vi "Send Inline Buffer.vi"(8 "error in (no error)":errorcluster, 10 "Inline Buffer Parameters":T1, 11 "Dispatcher Interface in":refnum<class "Dispatcher Interface.lvclass">) -> (0 "error out":errorcluster, 3 "Dispatcher Interface out":refnum<class "Dispatcher Interface.lvclass">)   [LabVIEW 2017, in "DSF Core.lvlib" / "Dispatcher Interface.lvclass"]
uses:
  Dispatcher Interface.lvclass
  C:/Git/DSF/Data Sharing Framework/Source/Core/Classes/Interfaces/Interface/Interface.lvclass
  Inline Buffer Parameters.ctl
  Command Data.ctl
  Command.ctl
  Parameters.ctl
  Interface/Interface.lvclass/Interface.ctl
  Response.ctl
  Write Dispatcher Command.vi
  Interface/Send Command.vi
  Interface/Write RT FIFO.vi
  Class Name.vi
  VIs/VI Name.vi
  Command Timeout.vi
  Read Dispatcher Response.vi
  Invalid Response Parameters.vi
  Invalid Response.vi
  Interface/Interface.lvclass
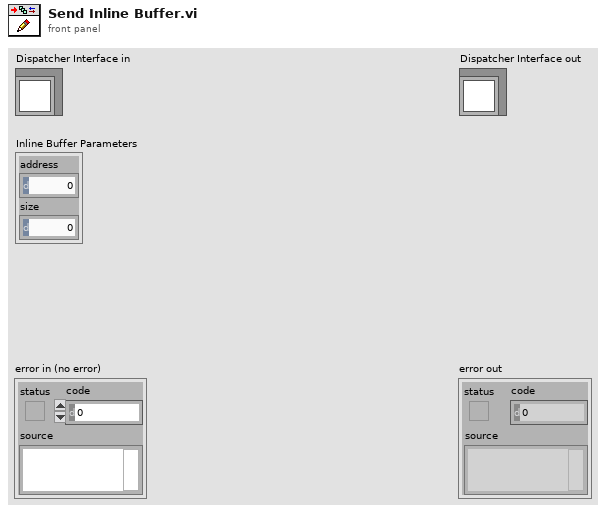
[diagram p1: front panel]
types:
  T1 = typedef "DSF Core.lvlib/Dispatcher Interface.lvclass/Inline Buffer Parameters.ctl" = cluster{"address":u64, "size":u64}
  T2 = typedef "DSF Core.lvlib/Dispatcher Interface.lvclass/Command.ctl" = enum8{"Rx", "Tx", "Set Inline Buffer", "Shutdown"}
  T3 = typedef "DSF Core.lvlib/Dispatcher Interface.lvclass/Parameters.ctl" = cluster{"arg1":u64, "arg2":u64}
  T4 = typedef "DSF Core.lvlib/Dispatcher Interface.lvclass/Command Data.ctl" = cluster{"Command":T2, "Parameters":T3}
  T5 = typedef "DSF Core.lvlib/Dispatcher Interface.lvclass/Response Data.ctl" = cluster{"Response":T6, "Parameters":T3}
  T6 = typedef "DSF Core.lvlib/Dispatcher Interface.lvclass/Response.ctl" = enum8{"General Ack", "Error", "Shutting Down"}
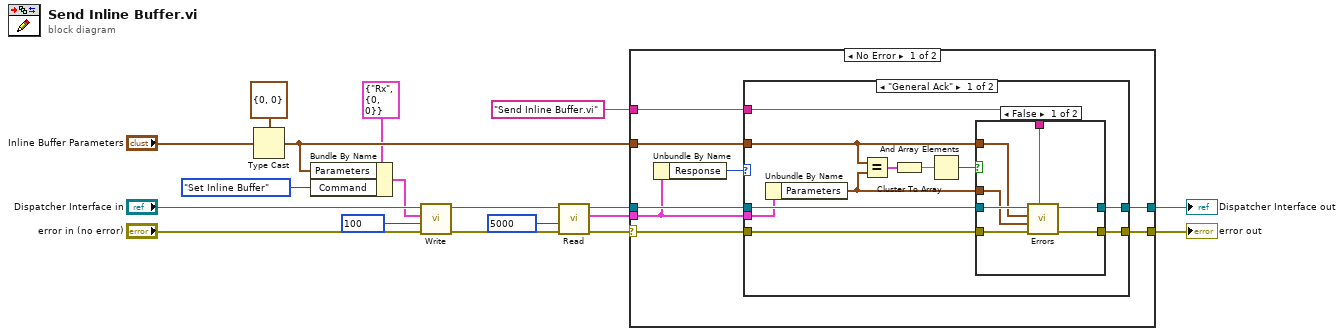
[diagram p0: block diagram]
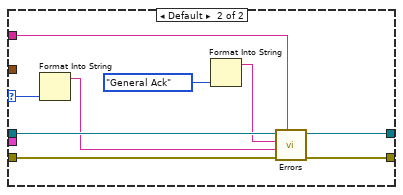
[diagram p3: hidden frame]
diagram:
  n1 = Type Cast(type=T3 {"arg1"=0, "arg2"=0} ("Parameters"), x="Inline Buffer Parameters") -> (*(type *) &x=w7:T3)
  n2 = Bundle By Name(cluster=T4 {"Command"=enum."Rx", "Parameters"={"arg1"=0, "arg2"=0}} ("command"), "Parameters"=w7, "Command"=Command."Set Inline Buffer") -> (w12:T4)
  n3 = call-poly "Write.vi"("error in (no error)"="error in (no error)", "timeout in ms (0)"=100, "command"=w12, "Dispatcher Interface in"="Dispatcher Interface in") -> ("error out"=w5:errorcluster, "Dispatcher Interface out"=w6:refnum<class "Dispatcher Interface.lvclass">)  [unwired: 6 in]
  n4 = call-poly "Read.vi"("error in (no error)"=w5, "timeout in ms (0)"=5000, "Dispatcher Interface in"=w6) -> ("error out"=w4:errorcluster, "response"=w8:T5, "Dispatcher Interface out"=w10:refnum<class "Dispatcher Interface.lvclass">)  [unwired: 5 in, 1 out]
  n5 = case shown="No Error" w4 {
    selector: w4 -> [w20 w56]
    tunnel: [w25 w56] -> w16
    tunnel: w7 -> [w24 _]
    tunnel: w10 -> [w23 w57]
    tunnel: [w22 w57] -> w15
    tunnel: w8 -> [w21 _]
    tunnel: "Send Inline Buffer.vi" ("error source vi name") -> [w19 _]
    frame No Error {
      n6 = Unbundle By Name(w21) -> ("Response"=w26:T6)
      n7 = case shown="\"General Ack\"" w26 {
        selector: w26 -> [_ w50]
        tunnel: w20 -> [w34 w54]
        tunnel: [w32 w52] -> w25
        tunnel: w24 -> [w29 _]
        tunnel: w23 -> [w31 w55]
        tunnel: [w33 w53] -> w22
        tunnel: w21 -> [w30 _]
        tunnel: w19 -> [w27 w51]
        frame "General Ack" {
          n8 = Unbundle By Name(w30) -> ("Parameters"=w28:T3)
          n9 = Equal?(x=w29, y=w28) -> (x = y?=w37:cluster{"arg1":bool, "arg2":bool})
          n10 = Cluster To Array(cluster=w37) -> (array=w36:bool[])
          n11 = And Array Elements(Boolean array=w36) -> (logical AND=w35:bool)
          n12 = case shown="False" w35 {
            tunnel: w34 -> [w43 w45]
            tunnel: w31 -> [w44 w46]
            tunnel: [w42 w46] -> w33
            tunnel: [w41 w45] -> w32
            tunnel: w29 -> [w39 _]
            tunnel: w28 -> [w40 _]
            tunnel: w27 -> [w38 _]
            frame False {
              n13 = call-poly "Errors.vi"("error source vi name"=w38, "error in (no error)"=w43, "actual parameters"=w40, "expected parameters"=w39, "Interface in"=w44) -> ("error out"=w41:errorcluster, "Interface out"=w42:refnum<class "Dispatcher Interface.lvclass">)  [unwired: 5 in]
            }
            frame True {
            }
          }
        }
        frame Default {
          n14 = Format Into String(w50) -> (resulting string=w49:string)  [unwired: 3 in, 1 out]
          n15 = Format Into String(Response."General Ack" ("expected response")) -> (resulting string=w47:string)  [unwired: 3 in, 1 out]
          n16 = call-poly "Errors.vi"("error source vi name"=w51, "error in (no error)"=w54, "actual response"=w49, "expected response"=w47, "Interface in"=w55) -> ("error out"=w52:errorcluster, "Interface out"=w53:refnum<class "Dispatcher Interface.lvclass">)  [unwired: 5 in]
        }
      }
    }
    frame Error {
      # "Incoming error. Pass through."
    }
  }
  "error out" <- w16
  "Dispatcher Interface out" <- w15
